vi "Write to Error Log File.vi"(8 "Error In":errorcluster, 10 "error in (no error)":errorcluster) -> (0 "Error Out":errorcluster)   [LabVIEW 2018]
panel:
  out "resulting string":string
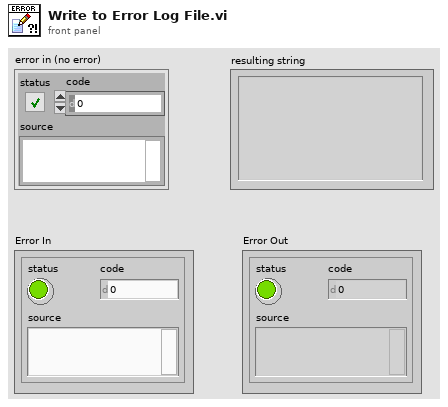
[diagram p1: front panel]
types:
  T1 = enum16{"open", "replace", "create", "open or create", "replace or create", "replace or create with confirmation"}
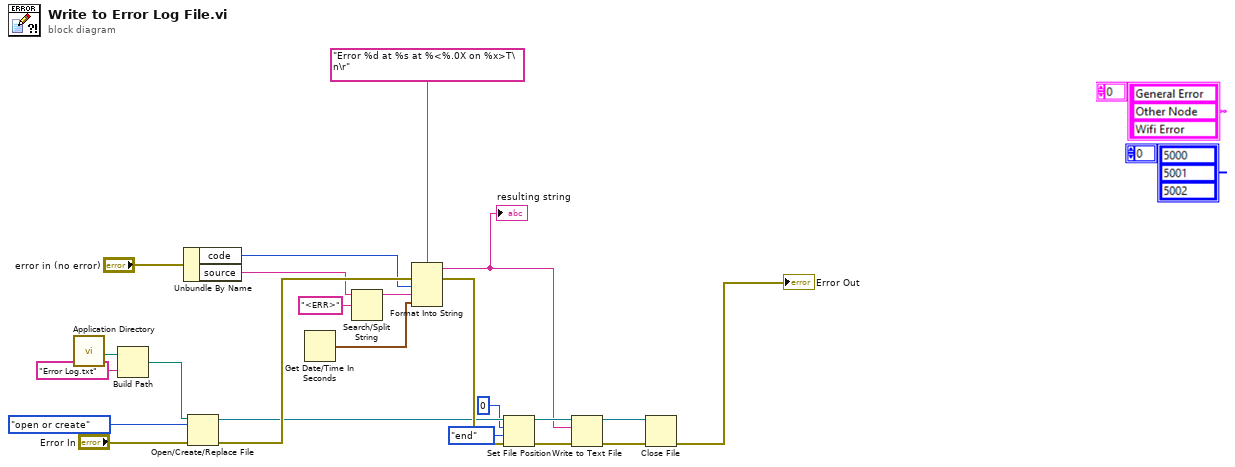
[diagram p0: block diagram]
diagram:
  n1 = call <vilib>:"Application Directory.vi"() -> ("Application Directory"=w19:path)
  n2 = Build Path(base path=w19, name or relative path="Error Log.txt") -> (appended path=w17:path)
  n3 = Unbundle By Name("error in (no error)") -> ("code"=w2:i32, "source"=w1:string)
  n4 = Open/Create/Replace File(file path (use dialog)=w17, error in="Error In", operation (0:open)=T1."open or create") -> (refnum out=w12:refnum<file>, error out=w20:errorcluster)  [unwired: 3 in, 1 out]
  n5 = Get Date/Time In Seconds() -> (seconds since 1Jan1904=w6:timestamp)
  n6 = Search/Split String(string=w1, search string/char (-)="<ERR>") -> (substring before match=w5:string)  [unwired: 1 in, 2 out]
  n7 = Format Into String(format string="Error %d at %s at %<%.0X on %x>T\n\r", error in=w20, w2, w5, w6) -> (resulting string=w7:string, error out=w22:errorcluster)  [unwired: 1 in]
  "resulting string" <- w7
  n8 = Set File Position(offset (in bytes) (0)=i64 0, refnum=w12, from (0:start)=enum16{"start", "end", "current"}."end", error in=w22) -> (refnum out=w11:refnum<file>, error out=w15:errorcluster)
  n9 = Write to Text File(file (use dialog)=w11, text=w7, error in=w15) -> (refnum out=w10:refnum<file>, error out=w14:errorcluster)  [unwired: 1 in, 1 out]
  n10 = Close File(refnum=w10, error in=w14) -> (error out=→"Error Out":errorcluster)  [unwired: 1 out]
